vi "Util_Trajectory_WriteFile_WayPoints.vi"(9 "UtilityWayPoints":T1[](array[typedef]) {"WEIGHT" format="%13.3f"; "ANGLE" format="%13.3f"; "Y" format="%13.3f"; "X" format="%13.3f"}, 11 "Byte Steam File In":refnum<file>) -> (0 "error out":errorcluster, 3 "Byte Steam File Out":refnum<file>)   [LabVIEW 2019, in "Trajectory_Library.lvlib"]
doc: "Internal routine to write trajectory waypoints to a file. \n\nParameters:\n - ByteStreamIn - File stream\n - Waypoints - waypoints to include in file comments (future)\n\nReturns:\n - ByteStreamOut - File stream\n - Error out - returned error cluster"
uses:
  Trajectory_Library.lvlib
  DISPLAY_WEIGHTED_WAYPOINT.ctl
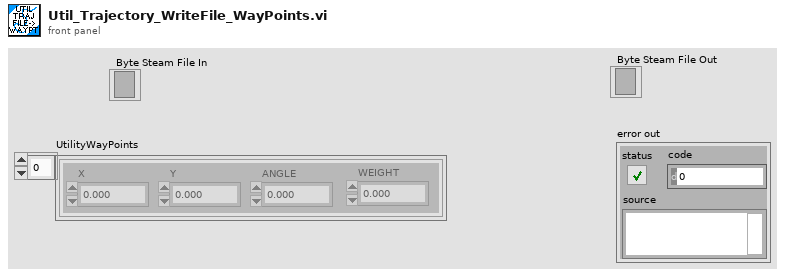
[diagram p1: front panel]
types:
  T1 = typedef "Trajectory_Library.lvlib/DISPLAY_WEIGHTED_WAYPOINT.ctl" = cluster{"X":dbl, "Y":dbl, "ANGLE":dbl, "WEIGHT":dbl}
  T2 = typedef "Trajectory_Library.lvlib/POSE2D.ctl" = cluster{"TRANSLATION":T3, "ROTATION":T4}
  T3 = typedef "Trajectory_Library.lvlib/TRANSLATION2D.ctl" = cluster{"X":dbl, "Y":dbl}
  T4 = typedef "Trajectory_Library.lvlib/ROTATION2D.ctl" = cluster{"VALUE":dbl, "COS":dbl, "SIN":dbl}
  T5 = typedef "Trajectory_Library.lvlib/TRANSFORM2D.ctl" = cluster{"TRANSLATION":T3, "ROTATION":T4}
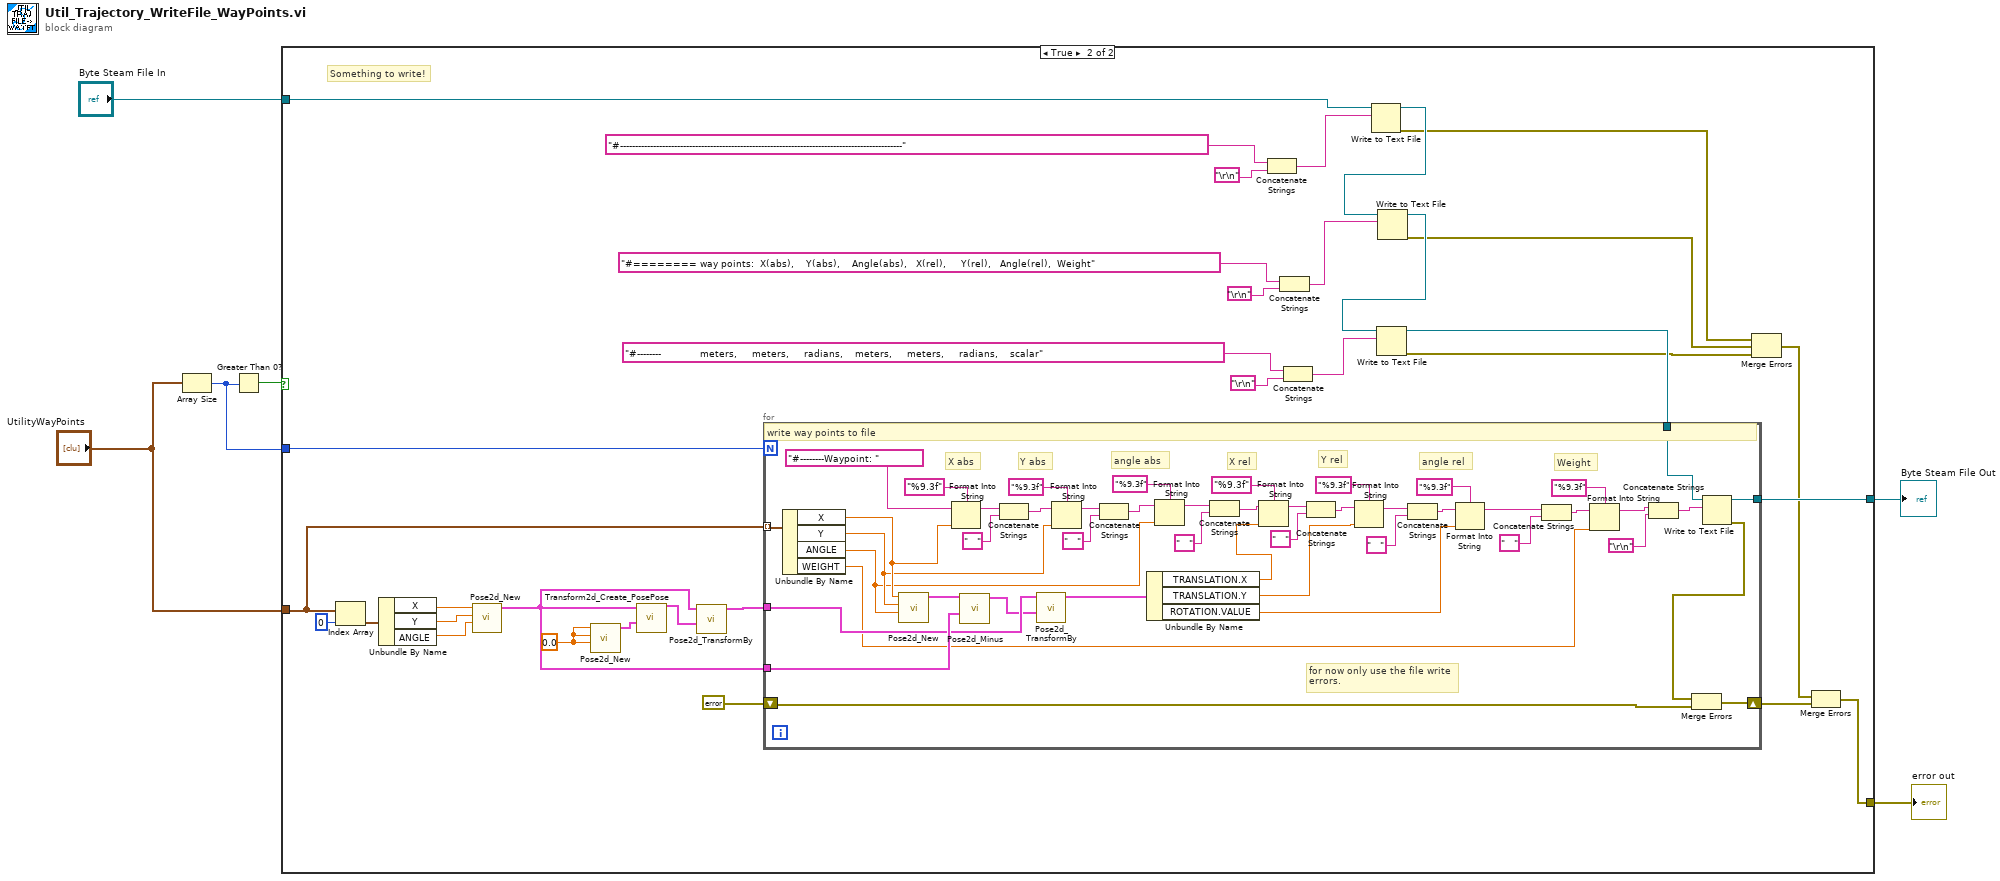
[diagram p0: block diagram]
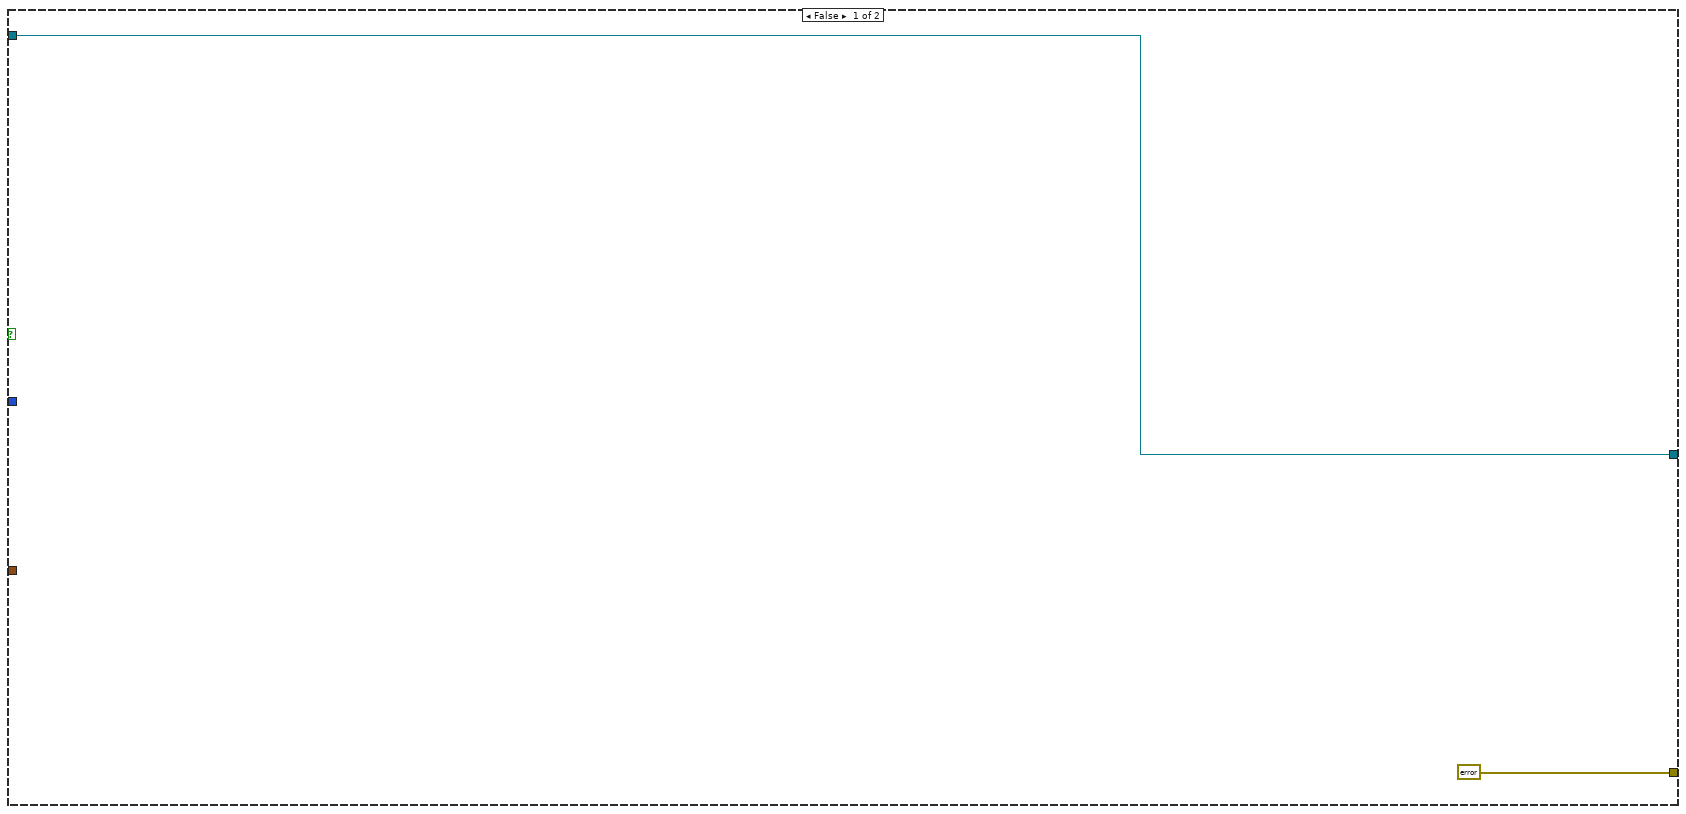
[diagram p2: hidden frame]
diagram:
  n1 = Array Size(array="UtilityWayPoints") -> (size(s)=w5:i32)
  n2 = Greater Than 0?(x=w5) -> (x > 0?=w3:bool)
  n3 = case shown="True" w3 {
    tunnel: [w8 w41] -> w6
    tunnel: w5 -> [_ w40]
    tunnel: "UtilityWayPoints" -> [_ w20]
    tunnel: "Byte Steam File In" -> [w8 w19]
    tunnel: [errorcluster {"status"=FALSE, "code"=0, "source"=""} ("error out") w9] -> w1
    frame False {
    }
    frame True {
      w39 = 0.0 ("X")
      # "Something to write!"
      n4 = Index Array(array=w20, index=0) -> (element=w34:T1)
      n5 = Unbundle By Name(w34) -> ("X"=w38:dbl, "Y"=w37:dbl, "ANGLE"=w36:dbl)
      n6 = call "Pose2d_New.vi"("Heading"=w36, "Y"=w37, "X"=w38) -> ("out POSe"=w30:T2)  [unwired: 8 in]
      n7 = call "Pose2d_New.vi"("Heading"=w39, "Y"=w39, "X"=w39) -> ("out POSe"=w33:T2)  [unwired: 8 in]
      n8 = call "Transform2d_Create_PosePose.vi"("last POSE"=w33, "initial POSE"=w30) -> ("TRANSFORM"=w32:T5)  [unwired: 9 in]
      n9 = call "Pose2d_TransformBy.vi"("other TRANSFORM"=w32, "in POSE"=w30) -> ("out POSE"=w31:T2)  [unwired: 9 in]
      n10 = Concatenate Strings("#----------------------------------------------------------------------------------------------" ("string"), "\r\n") -> (w21:string)
      n11 = Concatenate Strings("#======== way points:  X(abs),    Y(abs),    Angle(abs),   X(rel),     Y(rel),   Angle(rel),  Weight" ("string"), "\r\n") -> (w27:string)
      n12 = Concatenate Strings("#--------             meters,     meters,     radians,    meters,     meters,     radians,    scalar" ("string"), "\r\n") -> (w22:string)
      n13 = Write to Text File(file (use dialog)=w19, text=w21) -> (refnum out=w18:refnum<file>, error out=w15:errorcluster)  [unwired: 2 in, 1 out]
      n14 = Write to Text File(file (use dialog)=w18, text=w27) -> (refnum out=w17:refnum<file>, error out=w14:errorcluster)  [unwired: 2 in, 1 out]
      n15 = Write to Text File(file (use dialog)=w17, text=w22) -> (refnum out=w16:refnum<file>, error out=w13:errorcluster)  [unwired: 2 in, 1 out]
      n16 = for {
        N: w40 -> [_]
        tunnel: w20 -> [w78] mode=indexing
        tunnel: w16 -> [w76]
        tunnel: [w75] -> w41
        tunnel: w31 -> [w52]
        tunnel: w30 -> [w53]
        shift-right: [w50] -> w10
        shift-left: errorcluster {"status"=FALSE, "code"=0, "source"=""} ("error out") -> [w49]
        # "Weight"
        # "for now only use the file write\nerrors."
        # "angle rel"
        # "Y rel"
        # "X rel"
        # "angle abs"
        # "Y abs"
        # "X abs"
        # "write way points to file"
        n17 = Unbundle By Name(w78) -> ("X"=w61:dbl, "Y"=w60:dbl, "ANGLE"=w59:dbl, "WEIGHT"=w42:dbl)
        n18 = call "Pose2d_New.vi"("Heading"=w59, "Y"=w60, "X"=w61) -> ("out POSe"=w54:T2)  [unwired: 8 in]
        n19 = Format Into String(format string="%9.3f", initial string="#--------Waypoint: " ("string"), w61) -> (resulting string=w88:string)  [unwired: 1 in, 1 out]
        n20 = call "Pose2d_Minus.vi"("other TRANSFORM"=w53, "in POSE"=w54) -> ("outTRANSFORM"=w51:T5)  [unwired: 9 in]
        n21 = Concatenate Strings(w88, "   " ("string")) -> (w86:string)
        n22 = call "Pose2d_TransformBy.vi"("other TRANSFORM"=w51, "in POSE"=w52) -> ("out POSE"=w58:T2)  [unwired: 9 in]
        n23 = Format Into String(format string="%9.3f", initial string=w86, w60) -> (resulting string=w87:string)  [unwired: 1 in, 1 out]
        n24 = Concatenate Strings(w87, "   " ("string")) -> (w85:string)
        n25 = Unbundle By Name(w58) -> ("TRANSLATION.X"=w57:dbl, "TRANSLATION.Y"=w56:dbl, "ROTATION.VALUE"=w55:dbl)
        n26 = Format Into String(format string="%9.3f", initial string=w85, w59) -> (resulting string=w77:string)  [unwired: 1 in, 1 out]
        n27 = Concatenate Strings(w77, "   " ("string")) -> (w71:string)
        n28 = Format Into String(format string="%9.3f", initial string=w71, w57) -> (resulting string=w74:string)  [unwired: 1 in, 1 out]
        n29 = Concatenate Strings(w74, "   " ("string")) -> (w70:string)
        n30 = Format Into String(format string="%9.3f", initial string=w70, w56) -> (resulting string=w63:string)  [unwired: 1 in, 1 out]
        n31 = Concatenate Strings(w63, "   " ("string")) -> (w65:string)
        n32 = Format Into String(format string="%9.3f", initial string=w65, w55) -> (resulting string=w45:string)  [unwired: 1 in, 1 out]
        n33 = Concatenate Strings(w45, "   " ("string")) -> (w47:string)
        n34 = Format Into String(format string="%9.3f", initial string=w47, w42) -> (resulting string=w44:string)  [unwired: 1 in, 1 out]
        n35 = Concatenate Strings(w44, "\r\n") -> (w66:string)
        n36 = Write to Text File(file (use dialog)=w76, text=w66) -> (refnum out=w75:refnum<file>, error out=w48:errorcluster)  [unwired: 2 in, 1 out]
        n37 = Merge Errors(w48, w49) -> (w50:errorcluster)
      }
      n38 = Merge Errors(w15, w14, w13) -> (w12:errorcluster)
      n39 = Merge Errors(w12, w10) -> (w9:errorcluster)
    }
  }
  "error out" <- w1
  "Byte Steam File Out" <- w6
